vi "Write Buffer Configs.vi"(8 "error in (no error)":errorcluster, 10 "Buffer Configs":T1[](array[typedef]), 11 "Plugin in":refnum<class "Plugin.lvclass">) -> (0 "error out":errorcluster, 3 "Plugin out":refnum<class "Plugin.lvclass">)   [LabVIEW 2016, in "Plugin.lvclass"]
uses:
  Plugin.lvclass
  Typdefs/Buffer Configuration.ctl
  <vilib>/NI Veristand/VeriStand Data/Byte Buffer/Byte Buffer.Mapping.ctl
  <vilib>/NI Veristand/VeriStand Data/Typedefs/Typedefs.Data Types.ctl
  Typdefs/Decimation Factors.ctl
  Plugin.lvclass/Plugin.ctl
  <vilib>/NI Veristand/VeriStand Data/VeriStand Data.lvlib
  <vilib>/NI Veristand/VeriStand Data/Byte Buffer/Byte Buffer.lvclass
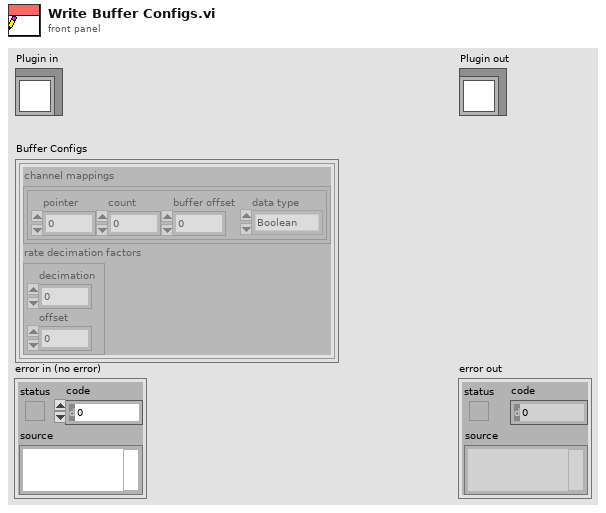
[diagram p1: front panel]
types:
  T1 = typedef "Buffer Configuration.ctl" = cluster{"channel mappings":T2[], "rate decimation factors":T4}
  T2 = typedef "VeriStand Data.lvlib/Byte Buffer.lvclass/Byte Buffer.Mapping.ctl" = cluster{"pointer":u64, "count":i64, "buffer offset":u64, "data type":T3}
  T3 = typedef "VeriStand Data.lvlib/Typedefs.Data Types.ctl" = enum16{"Boolean", "Single", "Double", "I8", "I16", "I32", "I64", "U8", "U16", "U32", "U64"}
  T4 = typedef "Decimation Factors.ctl" = cluster{"decimation":u16, "offset":u16}
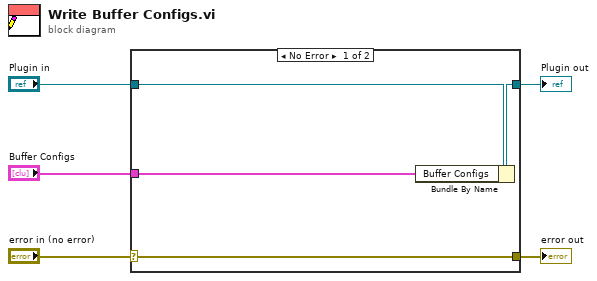
[diagram p0: block diagram]
diagram:
  n1 = case shown="No Error" "error in (no error)" {
    selector: "error in (no error)" -> [w9 w10]
    tunnel: [w9 w10] -> w4
    tunnel: [w7 w11] -> w2
    tunnel: "Plugin in" -> [w8 w11]
    tunnel: "Buffer Configs" -> [w6 _]
    frame No Error {
      n2 = Bundle By Name(cluster=w8, "Buffer Configs"=w6) -> (w7:refnum<class "Plugin.lvclass">)
    }
    frame Error {
    }
  }
  "error out" <- w4
  "Plugin out" <- w2
